vi "Configure Trigger.vi"(0 "VISA resource name":refnum<visa-resource-name>, 1 "Trigger Type (0: Continuous)":u16(ring) items=["Continuous", "Single", "Gate", "Segment Advance"], 2 "Trigger Source (0: Key)":u16(ring) items=["Key", "External", "Bus"], 5 "Modulation Format (0: Custom)":u16(ring) items=["Custom", "Dual Modulation", "Dual ARB"], 7 "Continuous Trigger Type (0: Free)":u16(ring) items=["Free", "Trigger", "Reset"], 9 "Retriggering Mode (0: ON)":u16(ring) items=["On", "Off", "Immediate"], 11 "error in (no error)":errorcluster, 12 "Gate Active (0: High)":u16(ring) items=["High", "Low"], 13 "Segment Advance Trigger Type (0: Continuous)":u16(ring) items=["Continuous", "Single"]) -> (4 "VISA resource name out":refnum<visa-resource-name>, 15 "error out":errorcluster)   [LabVIEW 2018, in "Agilent PSG MXG Series.lvlib"]
doc: "Configures the trigger source and trigger type for the specific modulation format.\n\n<B>Notes:</B>\n(1) This VI is valid only in E8267C, E8267D, N5162A, N5182A, N5172B, N5182B.\n\n(2) For E8267C, this VI is valid only when the instrument installs <B>Option 002</B> (Internal baseband generator) or <B>Option 602</B> (Digital bus baseband generator).\n\n(3) For E8267D, this VI is valid only when the instrument installs <B>Option 601</B> or <B>Option 602</B> (Internal baseband generator).\n\n(4) For N5162A and N5182A, this VI is valid only when the instrument installs <B>Option 651</B> or <B>Option 652</B> or <B>Option 654</B> (Internal baseband generator).\n\n(5) For N5172B and N5182B, custom and dual modulation is valid only when the instrument installs <B>Option 431</B>."
uses:
  Agilent PSG MXG Series.lvlib
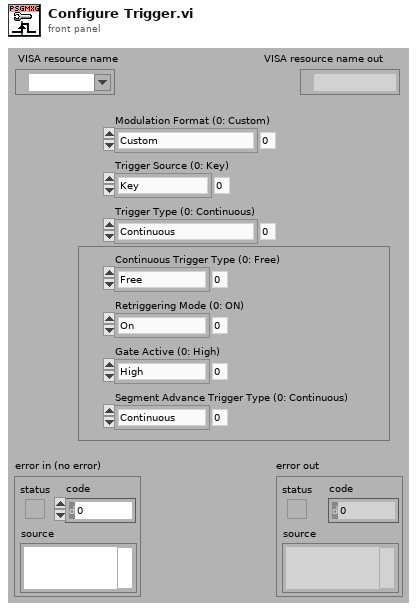
[diagram p1: front panel]
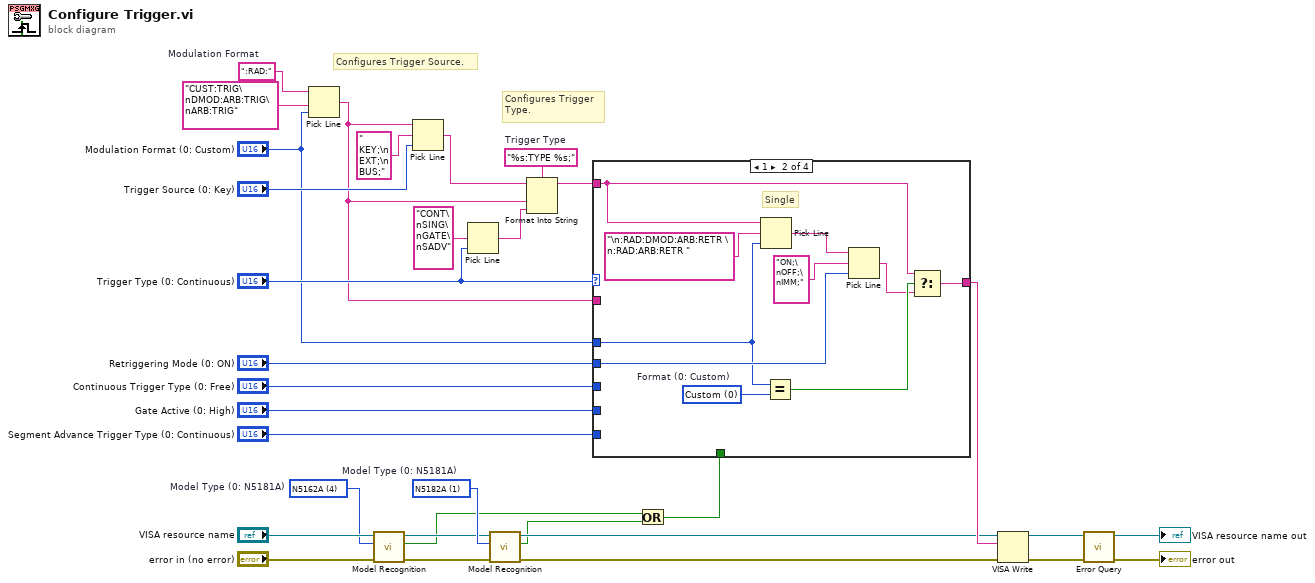
[diagram p0: block diagram]
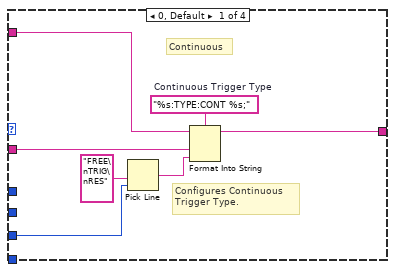
[diagram p2: hidden frame]
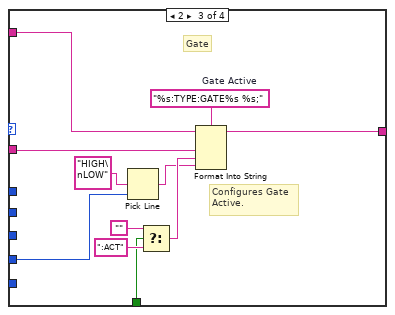
[diagram p3: hidden frame]
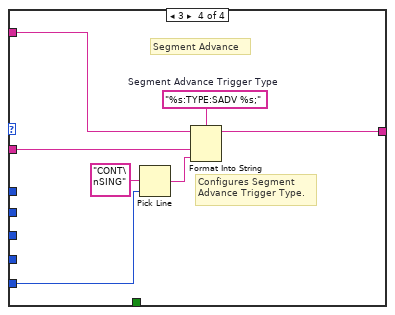
[diagram p4: hidden frame]
diagram:
  w4 = u16 4 items=["N5181A"=0, "N5182A"=1, "N5183A"=2, "N5161A"=3, "N5162A"=4, "E8241A"=5, "E8244A"=6, "E8251A"=7, "E8254A"=8, "E8247C"=10, "E8257C"=11, "E8267C"=12, "E8257D"=15, "E8267D"=16, "N5171B"=17, "N5172B"=18, "N5181B"=19, "N5182B"=20]  # Model Type (0: N5181A)
  w9 = u16 1 items=["N5181A"=0, "N5182A"=1, "N5183A"=2, "N5161A"=3, "N5162A"=4, "E8241A"=5, "E8244A"=6, "E8251A"=7, "E8254A"=8, "E8247C"=10, "E8257C"=11, "E8267C"=12, "E8257D"=15, "E8267D"=16, "N5171B"=17, "N5172B"=18, "N5181B"=19, "N5182B"=20]  # Model Type (0: N5181A)
  w27 = "%s:TYPE %s;"  # Trigger Type
  w32 = ":RAD:"  # Modulation Format
  # "Configures Trigger\nType."
  # "Configures Trigger Source."
  n1 = Pick Line(string ("")=w32, multi-line string="CUST:TRIG\nDMOD:ARB:TRIG\nARB:TRIG", line index="Modulation Format (0: Custom)") -> (output string=w23:string)
  n2 = call "Model Recognition.vi"("error in (no error)"="error in (no error)", "Model Type (0: N5181A)"=w4, "VISA resource name"="VISA resource name") -> ("error out"=w5:errorcluster, "Is Model Correct"=w2:bool, "VISA resource name out"=w7:refnum<visa-resource-name>)  [unwired: 6 out]
  n3 = Pick Line(string ("")=w23, multi-line string=" KEY;\n EXT;\n BUS;" ("Trigger Source"), line index="Trigger Source (0: Key)") -> (output string=w28:string)
  n4 = Pick Line(multi-line string="CONT\nSING\nGATE\nSADV", line index="Trigger Type (0: Continuous)") -> (output string=w26:string)  [unwired: 1 out]
  n5 = call "Model Recognition.vi"("error in (no error)"=w5, "Model Type (0: N5181A)"=w9, "VISA resource name"=w7) -> ("error out"=w15:errorcluster, "Is Model Correct"=w3:bool, "VISA resource name out"=w16:refnum<visa-resource-name>)  [unwired: 6 out]
  n6 = Format Into String(format string=w27, initial string=w28, w23, w26) -> (resulting string=w22:string)  [unwired: 1 in, 1 out]
  n7 = Or(x=w2, y=w3) -> (x .or. y?=w1:bool)
  n8 = case shown="1" "Trigger Type (0: Continuous)" {
    tunnel: w23 -> [w38 _ w59 w66]
    tunnel: w22 -> [w35 w41 w56 w62]
    tunnel: "Continuous Trigger Type (0: Free)" -> [w34 _ _ _]
    tunnel: "Gate Active (0: High)" -> [_ _ w57 _]
    tunnel: "Segment Advance Trigger Type (0: Continuous)" -> [_ _ _ w63]
    tunnel: [w33 w40 w55 w61] -> w19
    tunnel: "Retriggering Mode (0: ON)" -> [_ w46 _ _]
    tunnel: "Modulation Format (0: Custom)" -> [_ w45 _ _]
    tunnel: w1 -> [_ _ w50 _]
    frame 0, Default {
      w39 = "%s:TYPE:CONT %s;"  # Continuous Trigger Type
      # "Configures Continuous\nTrigger Type."
      # "Continuous"
      n9 = Pick Line(multi-line string="FREE\nTRIG\nRES", line index=w34) -> (output string=w37:string)  [unwired: 1 out]
      n10 = Format Into String(format string=w39, initial string=w35, w38, w37) -> (resulting string=w33:string)  [unwired: 1 in, 1 out]
    }
    frame 1 {
      w44 = u16 0 items=["Custom", "Dual Modulation", "Dual ARB"]  # Format (0: Custom)
      # "Single"
      n11 = Pick Line(string ("")=w41, multi-line string="\n:RAD:DMOD:ARB:RETR \n:RAD:ARB:RETR ", line index=w45) -> (output string=w48:string)
      n12 = Equal?(x=w45, y=w44) -> (x = y?=w43:bool)
      n13 = Pick Line(string ("")=w48, multi-line string="ON;\nOFF;\nIMM;", line index=w46) -> (output string=w42:string)
      n14 = Select(t=w41, s=w43, f=w42) -> (s? t:f=w40:string)
    }
    frame 2 {
      w60 = "%s:TYPE:GATE%s %s;"  # Gate Active
      # "Configures Gate\nActive."
      # "Gate"
      n15 = Pick Line(multi-line string="HIGH\nLOW", line index=w57) -> (output string=w53:string)  [unwired: 1 out]
      n16 = Select(t="", s=w50, f=":ACT") -> (s? t:f=w54:string)
      n17 = Format Into String(format string=w60, initial string=w56, w59, w54, w53) -> (resulting string=w55:string)  [unwired: 1 in, 1 out]
    }
    frame 3 {
      w67 = "%s:TYPE:SADV %s;"  # Segment Advance Trigger Type
      # "Configures Segment\nAdvance Trigger Type."
      # "Segment Advance"
      n18 = Pick Line(multi-line string="CONT\nSING", line index=w63) -> (output string=w65:string)  [unwired: 1 out]
      n19 = Format Into String(format string=w67, initial string=w62, w66, w65) -> (resulting string=w61:string)  [unwired: 1 in, 1 out]
    }
  }
  n20 = VISA Write(VISA resource name=w16, write buffer=w19, error in (no error)=w15) -> (VISA resource name out=w18:refnum<visa-resource-name>, error out=w17:errorcluster)  [unwired: 1 out]
  n21 = call "Error Query.vi"("error in (no error)"=w17, "VISA resource name"=w18) -> ("error out"=→"error out":errorcluster, "VISA resource name out"=→"VISA resource name out":refnum<visa-resource-name>)  [unwired: 8 out]
